vi "Close MDIF file.vi"(8 "error in (no error)":errorcluster, 11 "MDIF reference in":refnum<k24>) -> (0 "error out":errorcluster)   [LabVIEW 2023, in "NI_HFNetworkAnalysis.lvlib"]
doc: "Close reference to the MDIF File.\n\n<b>Note</b>\nUse <b>Save MDIF File.vi</b> to save the MDIF blocks in memory to file before closing the MDIF file reference."
uses:
  NI_HFNetworkAnalysis.lvlib
  C:/srd-semi-rfcal-software/AuxTools/STSRFFixtureCharactUtility/Source/Code Modules/Fixture/Dependencies/HFNetworkAnalysis/Support Files/NACE.Utils.Data.dll
  Support Files/NACE.Utils.Data.dll
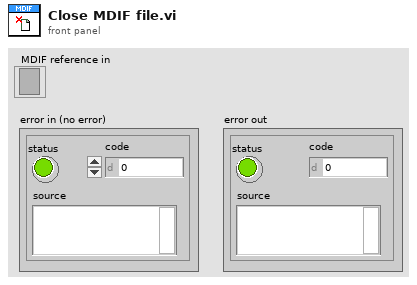
[diagram p1: front panel]
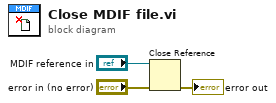
[diagram p0: block diagram]
diagram:
  n1 = Close Reference(reference="MDIF reference in", error in (no error)="error in (no error)") -> (error out=→"error out":errorcluster)
